vi "Ex_WiringPi_PWM.vi"(8 "error in (no error)":errorcluster) -> (0 "error out":errorcluster)   [LabVIEW 2014]
uses:
  vi.lib/Q-WaveSystems/QwaveSys Raspberry Pi for LabVIEW Home-Education/WiringPi/WiringPi Pin Mode.ctl
  vi.lib/Q-WaveSystems/QwaveSys Raspberry Pi for LabVIEW Home-Education/WiringPi/WiringPi GPIO TypeDef.ctl
  vi.lib/Q-WaveSystems/QwaveSys Raspberry Pi for LabVIEW Home-Education/QwaveSys Raspberry Pi Library.lvlib
panel:
  in  "WiringPi GPIO":T1=26 items=["SDA(I2C)-3"=8, "SCL(I2C)-5"=9, "MOSI(SPI)-19"=12, "MISO(SPI)-21"=13, "SCLK(SPI)-23"=14, "GPIO2-13"=2, "GPIO3-15"=3, "GPIO4-16"=4, "GPIO5-18"=5, "GPIO6-22"=6, "GPIO7-7"=7, "GPIO21-29"=21, "GPIO22-31"=22, "GPIO25-37"=25, "GPIO27-36"=27, "GPIO26(PWM0)-32"=26, "GPIO1(PWM0-12)"=1, "GPIO23(PWM1)-14"=23, "GPIO24(PWM1)-35"=24, "TXD(UART)-8"=15, "RXD(UART)-10"=16, "GPIO10(CE0-SPI)-24"=10, "GPPI11(CE1)-SPI)-26"=11, "GPIO28(PCM_DIN)36"=28, "GPIO29(PCM_DOUT)40"=29]
  out "PWM Output":u16(knob)=862 scale=0.0..1023.0
  in  "Pin Mode":T2=enum."PWM_OUTPUT"
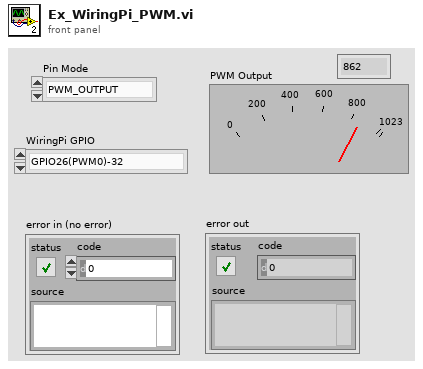
[diagram p1: front panel]
types:
  T1 = typedef "QwaveSys Raspberry Pi Library.lvlib/WiringPi GPIO TypeDef.ctl" = u8
  T2 = typedef "QwaveSys Raspberry Pi Library.lvlib/WiringPi Pin Mode.ctl" = enum8{"INPUT", "OUTPUT", "PWM_OUTPUT", "GPIO_CLOCK", "SOFT_PWM_OUTPUT", "SOFT_TONE_OUTPUT", "PWM_TONE_OUTPUT"}
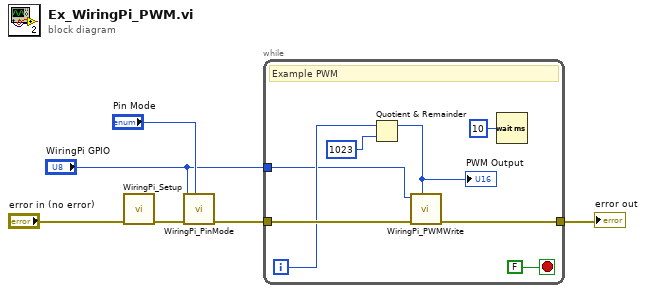
[diagram p0: block diagram]
diagram:
  n1 = call "WiringPi_Setup.vi"("error in (no error)"="error in (no error)") -> ("error out"=w5:errorcluster)  [unwired: 10 in]
  n2 = call "WiringPi_PinMode.vi"("Pin Mode"="Pin Mode", "error in (no error)"=w5, "WiringPi GPIO"="WiringPi GPIO") -> ("error out"=w4:errorcluster)  [unwired: 8 in]
  n3 = while {
    tunnel: w4 -> [w12]
    tunnel: [w11] -> w2
    tunnel: "WiringPi GPIO" -> [w7]
    i -> [w9]
    stop <- FALSE stop-if-true
    # "Example PWM"
    n4 = Quotient & Remainder(x=w9, y=1023) -> (x-y*floor(x/y)=w8:i32)  [unwired: 1 out]
    "PWM Output" <- w8
    n5 = call "WiringPi_PWMWrite.vi"("Value"=w8, "error in (no error)"=w12, "WiringPi GPIO"=w7) -> ("error out"=w11:errorcluster)  [unwired: 8 in]
    n6 = Wait (ms)(milliseconds to wait=u32 10) -> ()  [unwired: 1 out]
  }
  "error out" <- w2
